vi "Get Contact(ID).vi"(8 "error in (no error)":errorcluster, 11 "ID":u32) -> (0 "error out":errorcluster, 2 "Contact":T1, 3 "ID dup":u32)   [LabVIEW 2014, in "Contact Data.lvlib"]
doc: "Retrieves a single contact by ID from the address book data store."
uses:
  Contact Data.lvlib
  Contact.ctl
  Position.ctl
  Controls.ctl
  DestinationCluster.ctl
  DesinationControls.ctl
  Command.ctl
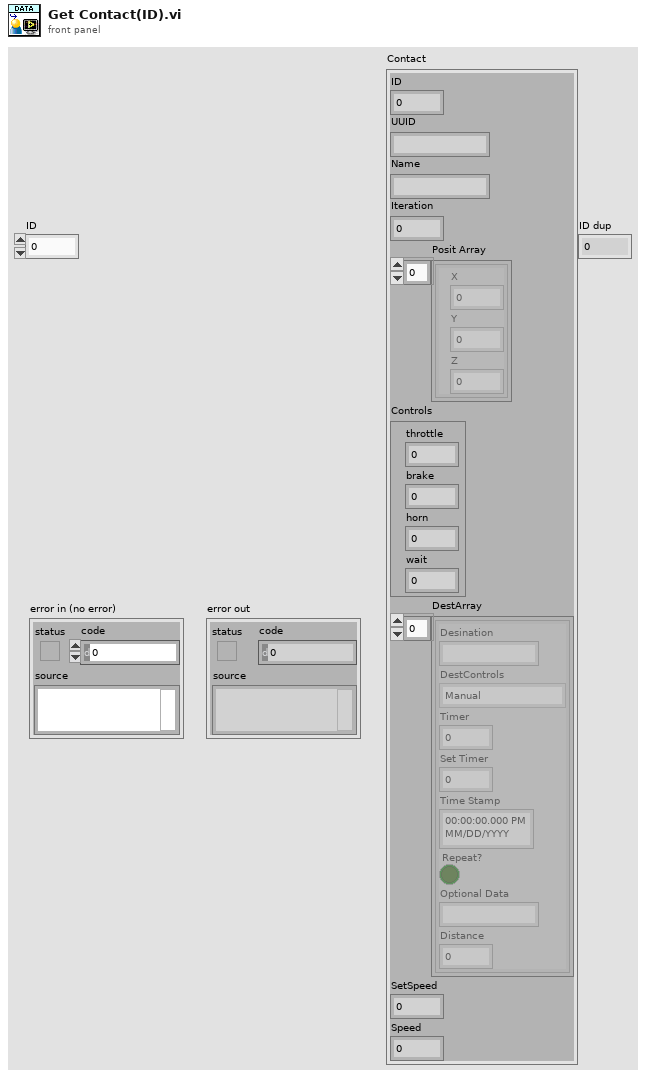
[diagram p1: front panel]
types:
  T1 = typedef "Contact Data.lvlib/Contact.ctl" = cluster{"ID":u32, "UUID":string, "Name":string, "Iteration":i32, "Posit Array":T2[], "Controls":T3, "DestArray":T4[], "SetSpeed":dbl, "Speed":dbl}
  T2 = typedef "Contact Data.lvlib/Position.ctl" = cluster{"X":dbl, "Y":dbl, "Z":dbl}
  T3 = typedef "Contact Data.lvlib/Controls.ctl" = cluster{"throttle":dbl, "brake":dbl, "horn":dbl, "wait":dbl}
  T4 = typedef "Contact Data.lvlib/DestinationCluster.ctl" = cluster{"Desination":string, "DestControls":T5, "Timer":u32, "Set Timer":u32, "Time Stamp":timestamp, "Repeat?":bool, "Optional Data":string, "Distance":dbl}
  T5 = typedef "Contact Data.lvlib/DesinationControls.ctl" = enum16{"Tracker", "Manual", "Stop", "Station DateTime", "Station Timer", "Maintain"}
  T6 = typedef "Contact Data.lvlib/Command.ctl" = enum16{"Set All Contacts", "Load", "Save", "Get All Data", "Get Single Data (ID)", "Get Single Data", "Set Position", "Set Destinations", "Set Controls", "Remove Single Data", "Remove UUID Contact", "Set Single ALL", "Is Data Modified", "Import Data"}
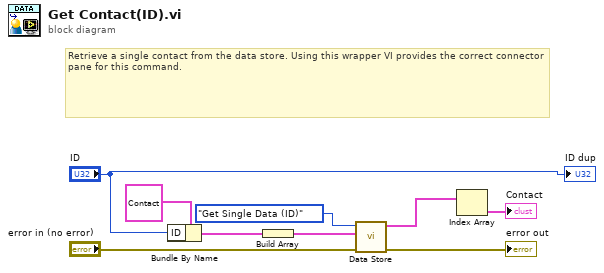
[diagram p0: block diagram]
diagram:
  # "Retrieve a single contact from the data store. Using this wrapper VI provides the correct connector pane for this command."
  n1 = Bundle By Name(cluster=T1 {"ID"=0, "UUID"="", "Name"="", "Iteration"=0, "Posit Array"=[], "Controls"={"throttle"=0.0, "brake"=0.0, "horn"=0.0, "wait"=0.5}, "DestArray"=[], "SetSpeed"=0.0, "Speed"=0.0} ("Contact"), "ID"="ID") -> (w8:T1)
  n2 = Build Array(w8) -> (w3:T1[])
  n3 = call "Data Store.vi"("error in (no error)"="error in (no error)", "Contact in"=w3, "Command"=Command."Get Single Data (ID)") -> ("error out"=→"error out":errorcluster, "Contacts out"=w4:T1[])  [unwired: 6 in, 1 out]
  n4 = Index Array(array=w4) -> (element=→"Contact":T1)  [unwired: 1 in]
  "ID dup" <- "ID"
